vi "create default alias.vi"(8 "error in":errorcluster, 11 "shared memory module configuration":refnum<class "Shared Memory Configuration.lvclass">) -> (0 "error out":errorcluster, 2 "default alias":string, 3 "shared memory module configuration out":refnum<class "Shared Memory Configuration.lvclass">)   [LabVIEW 2013, in "Shared Memory Configuration.lvclass"]
uses:
  Shared Memory Configuration.lvclass
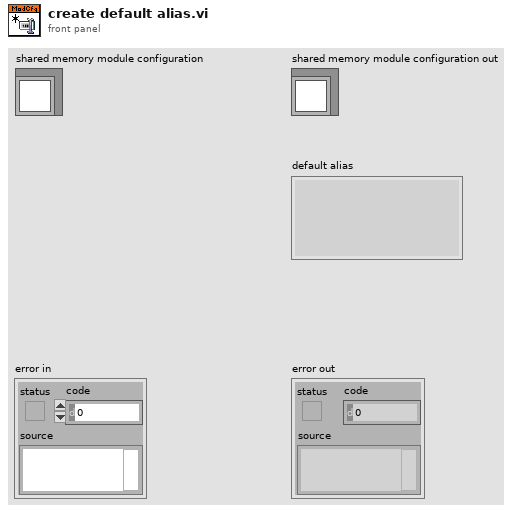
[diagram p1: front panel]
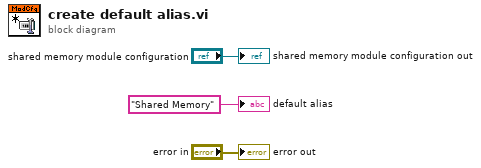
[diagram p0: block diagram]
diagram:
  "error out" <- "error in"
  "shared memory module configuration out" <- "shared memory module configuration"
  "default alias" <- "Shared Memory" ("search string")
